vi "Trapezoid Applier.vi"(8 "Intended Position":dbl=0.5, 9 "Distance Decrease":dbl, 10 "Distance to Setpoint":dbl, 11 "MotorControlDevRef in":T1) -> (2 "charted V":cluster{"Sensor Velocity":dbl, "Numeric":dbl}[](array[cluster]), 3 "Sensor Position out":dbl)   [LabVIEW 2023]
uses:
  <vilib>/Rock Robotics/WPI/MotorControl/WPI_MotorControlDeviceRef.ctl
  <vilib>/Rock Robotics/WPI/MotorControl/WPI_MotorControlType.ctl
  <vilib>/Rock Robotics/SystemInterfaces/DIO/FPGA_DIOPWMChannel.ctl
  <vilib>/Rock Robotics/WPI/PWM/WPI_PWMDeadband.ctl
  <vilib>/Rock Robotics/SystemInterfaces/DIO/FPGA_DIOChannel.ctl
  <vilib>/Rock Robotics/WPI/ThirdParty/REV Robotics/REVLib/Typedef/Spark MAX Control Type.ctl
  <vilib>/Rock Robotics/WPI/ThirdParty/REV Robotics/REVLib/Typedef/SPARK Closed Loop Slot.ctl
  <vilib>/Rock Robotics/WPI/ThirdParty/REV Robotics/REVLib/SubVI/Public/SPARK Get Encoder Status Position.vi
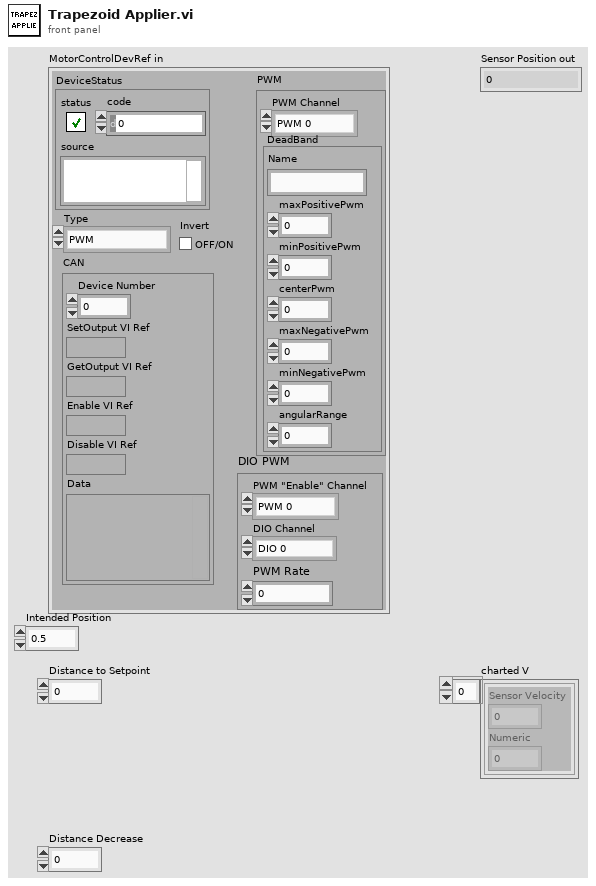
[diagram p1: front panel]
types:
  T1 = typedef "WPI_MotorControlDeviceRef.ctl" = cluster{"DeviceStatus":errorcluster, "Type":T2, "PWM":cluster{"PWM Channel":T3, "DeadBand":T4}, "CAN":cluster{"Device Number":u8, "SetOutput VI Ref":variant, "GetOutput VI Ref":variant, "Enable VI Ref":variant, "Disable VI Ref":variant, "Data":variant}, "Invert":bool, "DIO PWM":cluster{"PWM \"Enable\" Channel":T3, "DIOChannel":T5, "PWM Rate":dbl}}
  T2 = typedef "WPI_MotorControlType.ctl" = enum16{"PWM", "CAN", "DIO PWM"}
  T3 = typedef "FPGA_DIOPWMChannel.ctl" = enum8{"PWM 0", "PWM 1", "PWM 2", "PWM 3", "PWM 4", "PWM 5", "PWM 6", "PWM 7", "PWM 8", "PWM 9", "PWM MXP 0", "PWM MXP 1", "PWM MXP 2", "PWM MXP 3", "PWM MXP 4", "PWM MXP 5", "PWM MXP 6", "PWM MXP 7", "PWM MXP 8", "PWM MXP 9", "Invalid"}
  T4 = typedef "WPI_PWMDeadband.ctl" = cluster{"Name":string, "maxPositivePwm":i32, "minPositivePwm":i32, "centerPwm":i32, "maxNegativePwm":i32, "minNegativePwm":i32, "angularRange":u16}
  T5 = typedef "FPGA_DIOChannel.ctl" = enum8{"DIO 0", "DIO 1", "DIO 2", "DIO 3", "DIO 4", "DIO 5", "DIO 6", "DIO 7", "DIO 8", "DIO 9", "DIO MXP 0", "DIO MXP 1", "DIO MXP 2", "DIO MXP 3", "DIO MXP 4", "DIO MXP 5", "DIO MXP 6", "DIO MXP 7", "DIO MXP 8", "DIO MXP 9", "DIO MXP 10", "DIO MXP 11", "DIO MXP 12", "DIO MXP 13", "DIO MXP 14", "DIO MXP 15", "SPI Port CS1", "SPI Port CS2", "SPI Port CS3", "SPI Port MISO", "SPI Port MOSI", "Invalid"}
  T6 = typedef "SPARK Closed Loop Slot.ctl" = u16
  T7 = typedef "Spark MAX Control Type.ctl" = enum16{"Percent VBus", "Voltage", "Velocity", "Position", "Smart Motion", "Current", "Smart Velocity", "MAXMotion Position", "MAXMotion Velocity"}
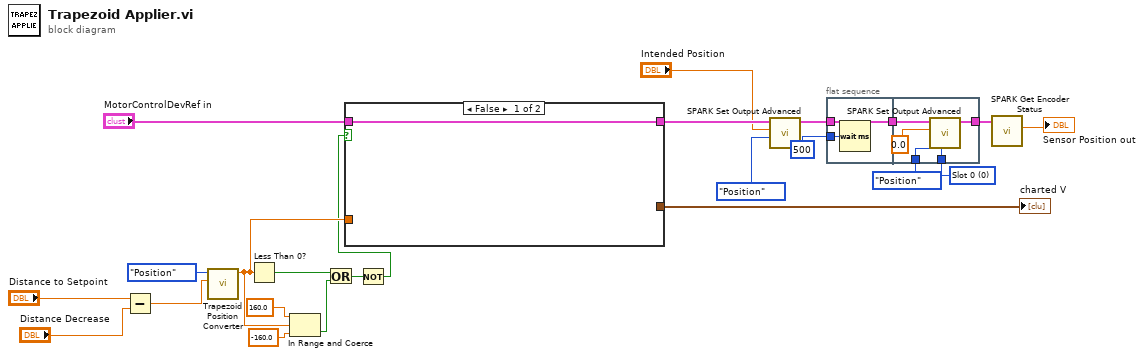
[diagram p0: block diagram]
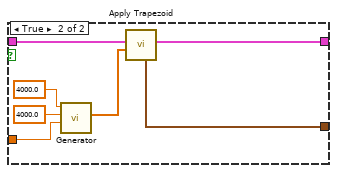
[diagram p2: hidden frame]
diagram:
  w1 = T6 0 items=["Slot 0", "Slot 1", "Slot 2", "Slot 3"] ("Closed Loop Slot")
  n1 = Subtract(x="Distance to Setpoint", y="Distance Decrease") -> (x-y=w7:dbl)
  n2 = call "Trapezoid Position Converter.vi"("Distance"=w7, "Initial Parameter"=enum16{"Position", "Trapezoid Distance"}."Position") -> ("Transformed Distance"=w21:dbl)  [unwired: 9 in]
  n3 = Less Than 0?(x=w21) -> (x < 0?=w15:bool)
  n4 = In Range and Coerce(upper limit=160.0, x=w21, lower limit=-160.0) -> (In Range?=w17:bool)  [unwired: 1 out]
  n5 = Or(x=w15, y=w17) -> (x .or. y?=w16:bool)
  n6 = Not(x=w16) -> (.not. x?=w20:bool)
  n7 = case shown="False" w20 {
    tunnel: "MotorControlDevRef in" -> [w24 w29]
    tunnel: [w24 w27] -> w12
    tunnel: w21 -> [_ w26]
    tunnel: [_ w25] -> w23
    frame False {
    }
    frame True {
      n8 = call "Generator.vi"("Distance"=w26, "Velocity Max"=4000.0 ("Acceleration Max"), "Acceleration Max"=4000.0) -> ("Velocity values"=w28:dbl[])  [unwired: 7 in, 1 out]
      n9 = call "Apply Trapezoid.vi"("Velocity values"=w28, "MotorControlDeviceRef in"=w29) -> ("MotorControlDevRef out"=w27:T1, "charted V"=w25:cluster{"Sensor Velocity":dbl, "Numeric":dbl}[])  [unwired: 6 in, 2 out]
    }
  }
  "charted V" <- w23
  n10 = call <vilib>:"SPARK Set Output Advanced.vi"("Control Mode"=Spark_MAX_Control_Type."Position", "Setpoint"="Intended Position", "MotorControlDevRef"=w12) -> ("MotorControlDevRef"=w6:T1)  [unwired: 7 in, 1 out]
  n11 = flat-sequence {
    tunnel: w6 -> [w33]
    tunnel: [w33] -> w5
    tunnel: u32 500 ("milliseconds to wait") -> [w32]
    tunnel: w5 -> [w38]
    tunnel: Spark_MAX_Control_Type."Position" ("Control Mode") -> [w36]
    tunnel: [w35] -> w2
    tunnel: w1 -> [w34]
    frame #0 {
      n12 = Wait (ms)(milliseconds to wait=w32) -> ()  [unwired: 1 out]
    }
    frame #1 {
      n13 = call <vilib>:"SPARK Set Output Advanced.vi"("Closed Loop Slot"=w34, "Control Mode"=w36, "Setpoint"=0.0, "MotorControlDevRef"=w38) -> ("MotorControlDevRef"=w35:T1)  [unwired: 6 in, 1 out]
    }
  }
  n14 = call-poly <vilib>:"SPARK Get Encoder Status.vi"("MotorControlDevRef in"=w2) -> ("Sensor Position"=→"Sensor Position out":dbl)  [unwired: 7 in, 3 out]
